vi "classify error.vi"(8 "error to classify":errorcluster, 11 "Modbus Slave runtime in":refnum<class "Modbus Module runtime.lvclass">) -> (0 "classified error":errorcluster, 2 "error classification":T1, 3 "Modbus Slave runtime out":refnum<class "Modbus Module runtime.lvclass">)   [LabVIEW 2013, in "Modbus Module runtime.lvclass"]
doc: "Allows a module to classify an error generated at any point during execution. This <b>error classification</b> can then be used by calling code to determine if execution can continue. In addition, this function can be used to allow a component to clear an error, convert an error to a warning, or attempt to recover from an error. Recovery may be attempted only if <b>attempt recovery?</b> is true.Platypus Framework 1.0.1.65\nNI Systems Engineering - National Instruments"
uses:
  Modbus Module runtime.lvclass
  <vilib>/NI/Tag Bus Module Framework/runtime/error classification.ctl
  <vilib>/NI/Tag Bus Module Framework/runtime/TBM module execution interface.lvclass
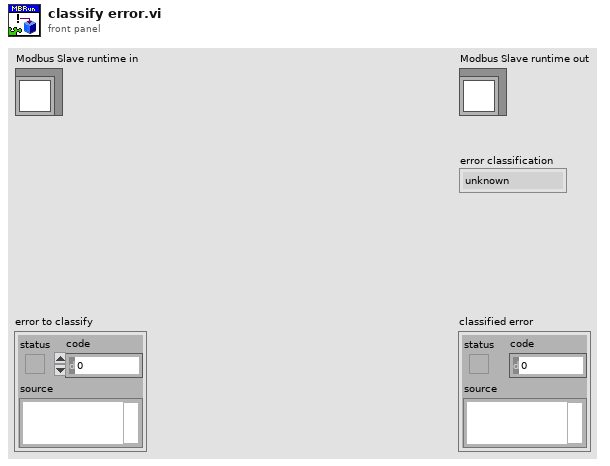
[diagram p1: front panel]
types:
  T1 = typedef "TBM module execution interface.lvclass/error classification.ctl" = enum16{"unknown", "none", "trivial", "recoverable", "critical"}
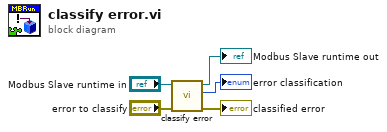
[diagram p0: block diagram]
diagram:
  n1 = call-parent "classify error.vi"("error to classify"="error to classify", "module in"="Modbus Slave runtime in") -> ("classified error"=→"classified error":errorcluster, "error classification"=→"error classification":T1, "module out"=→"Modbus Slave runtime out":refnum<class "Modbus Module runtime.lvclass">)  [unwired: 7 in]
